vi "For循环强制跳出.vi"() -> ()   [LabVIEW 2023]
panel:
  out "循环次数":i32
  in  "Array":string[](array[string])
  # "For 循环强制跳出"
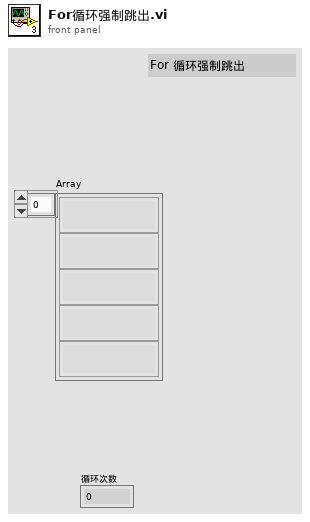
[diagram p1: front panel]
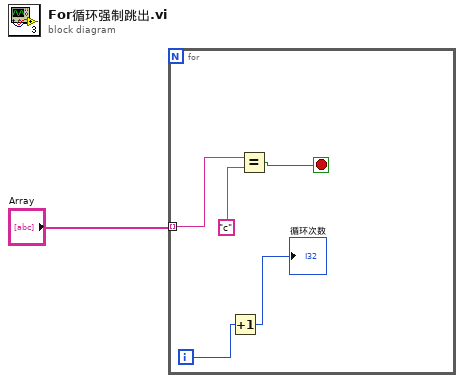
[diagram p0: block diagram]
diagram:
  n1 = for {
    tunnel: "Array" -> [w6] mode=indexing
    i -> [w3]
    stop <- w4 stop-if-true
    n2 = Increment(x=w3) -> (x+1=→"循环次数":i32)
    n3 = Equal?(x=w6, y="c") -> (x = y?=w4:bool)
  }
